vi "TomsToolsDocumentationTool_Item_OnCommand.vi"(10 "Command ID":string, 11 "Object":T1) -> ()   [LabVIEW 2015]
uses:
  Source Code/Model Messages/Add VI from File Msg/Add VI from File Msg.lvclass
  <resource>/Framework/Providers/API/ItemRef.ctl
panel:
  out "error out":errorcluster
  in  "error in":errorcluster
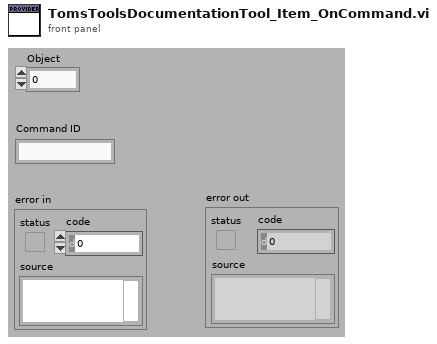
[diagram p1: front panel]
types:
  T1 = typedef "ItemRef.ctl" = u64
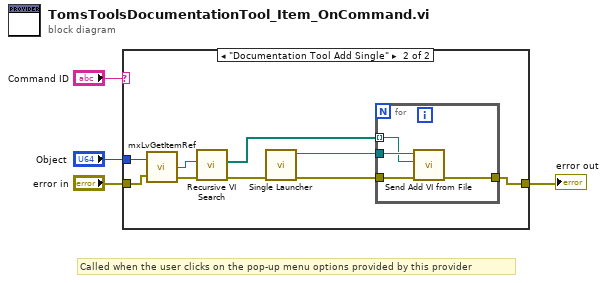
[diagram p0: block diagram]
diagram:
  # "Called when the user clicks on the pop-up menu options provided by this provider"
  n1 = case shown="\"Documentation Tool Add Single\"" "Command ID" {
    tunnel: "error in" -> [w5 w14]
    tunnel: [w5 w11] -> w2
    tunnel: "Object" -> [_ w13]
    frame Default {
    }
    frame "Documentation Tool Add Single" {
      n2 = call <resource>:"mxLvGetItemRef.vi"("Item"=w13, "error in"=w14) -> ("Item Refnum"=w6:refnum<vi>, "error out"=w10:errorcluster)  [unwired: 1 out]
      n3 = call "Recursive VI Search.vi"("error in (no error)"=w10, "Project Item"=w6) -> ("error out"=w9:errorcluster, "VI Paths"=w7:path[])  [unwired: 8 in]
      n4 = call "Single Launcher.vi"("error in (no errors)"=w9) -> ("error out"=w8:errorcluster, "Documentation Tool Model"=w12:refnum<class "Message Enqueuer.lvclass">)  [unwired: 9 in]
      n5 = for {
        tunnel: w12 -> [w18]
        tunnel: [w17] -> w11
        tunnel: w7 -> [w16] mode=indexing
        tunnel: w8 -> [w15]
        n6 = call "Send Add VI from File.vi"("error in (no error)"=w15, "VI Path"=w16, "Message Enqueuer"=w18) -> ("error out"=w17:errorcluster)  [unwired: 7 in, 1 out]
      }
    }
  }
  "error out" <- w2
